vi "Compute_Anomaly_Map.vi"(8 "error in":errorcluster, 9 "Gaussian Blur":T1={"Kernel_Size"=33, "sigma"=4.0}, 10 "input img size":i32[](array[numeric]), 11 "patch scores [bs,h,w]":sgl[][][](array[numeric])) -> (0 "error IO":errorcluster, 3 "anomaly map":sgl[][][](array[numeric]))   [LabVIEW 2020]
uses:
  API/Controls/Gaussian_Blur.ctl
  <vilib>/addons/Multicore Analysis and Sparse Matrix/Signal Operation/_sigop/Convolution_Output Size.ctl
  <vilib>/addons/Multicore Analysis and Sparse Matrix/Signal Operation/_sigop/Algorithm Domain.ctl
  <vilib>/Ngene/Deep Learning Toolkit/Toolkit/NN_Layers/Layers/Input/subVIs/Augmentation/Blur/SubVI/Gauss_Function.vi
  <vilib>/Utility/High Resolution Relative Seconds.vi
  Intrplt_Get_Dest_Coords.vi
  <vilib>/addons/Multicore Analysis and Sparse Matrix/Signal Operation/_sigop/2D Convolution (SGL).vi
  <vilib>/Ngene/Deep Learning Toolkit/Toolkit/Deep_Learning_Toolkit_by_Ngene.lvlib
  <vilib>/addons/Multicore Analysis and Sparse Matrix/Signal Operation/NI_MASM_SigOperation.lvlib
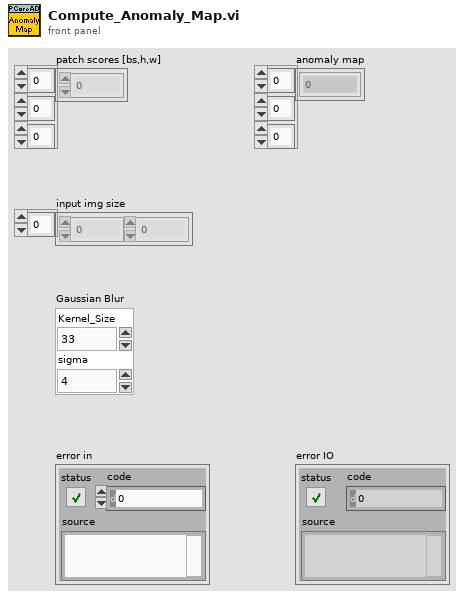
[diagram p1: front panel]
types:
  T1 = typedef "Gaussian_Blur.ctl" = cluster{"Kernel_Size":i32, "sigma":sgl}
  T2 = typedef "NI_MASM_SigOperation.lvlib/Convolution_Output Size.ctl" = i32
  T3 = typedef "NI_MASM_SigOperation.lvlib/Algorithm Domain.ctl" = i32
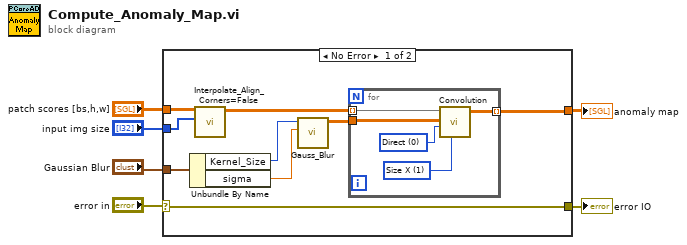
[diagram p0: block diagram]
diagram:
  n1 = case shown="No Error" "error in" {
    selector: "error in" -> [w15 w21]
    tunnel: "input img size" -> [w13 _]
    tunnel: [w7 _] -> w3
    tunnel: "patch scores [bs,h,w]" -> [w14 _]
    tunnel: [w15 w21] -> w4
    tunnel: "Gaussian Blur" -> [w10 _]
    frame No Error {
      n2 = Unbundle By Name(w10) -> ("Kernel_Size"=w9:i32, "sigma"=w8:sgl)
      n3 = call "Interpolate_Align_Corners=False.vi"("target Dims"=w13, "Array"=w14) -> ("Out"=w11:sgl[][][])  [unwired: 8 in, 1 out]
      n4 = call <vilib>:"Gauss_Blur.vi"("sigma"=w8, "Kernel_Size"=w9) -> ("Kernel"=w12:sgl[][])  [unwired: 9 in]
      n5 = for {
        tunnel: [w20] -> w7 mode=indexing
        tunnel: w12 -> [w18]
        tunnel: w11 -> [w19] mode=indexing
        w16 = T2 1 items=["Full", "Size X", "Compact"] ("output size")
        w17 = T3 0 items=["Direct", "Frequency Domain"] ("algorithm")
        n6 = call-poly <vilib>:"Convolution.vi"("output size"=w16, "algorithm"=w17, "Y"=w18, "X"=w19) -> ("X * Y"=w20:sgl[][])  [unwired: 6 in, 1 out]
      }
    }
    frame Error {
    }
  }
  "anomaly map" <- w3
  "error IO" <- w4
